vi "Read channels.vi"(8 "error in":errorcluster, 11 "Tag Bus Web Interface configuration in":refnum<class "Tag Bus Web Interface configuration.lvclass">) -> (0 "error out":errorcluster, 2 "channels":refnum<class "TBM channel.lvclass">[](array[class]), 3 "Tag Bus Web Interface configuration out":refnum<class "Tag Bus Web Interface configuration.lvclass">)   [LabVIEW 2013, in "Tag Bus Web Interface configuration.lvclass"]
uses:
  Tag Bus Web Interface configuration.lvclass
  <vilib>/NI/Tag Bus Module Framework/channel/TBM channel.lvclass
  Tag Bus Web Interface configuration.lvclass/Tag Bus Web Interface configuration.ctl
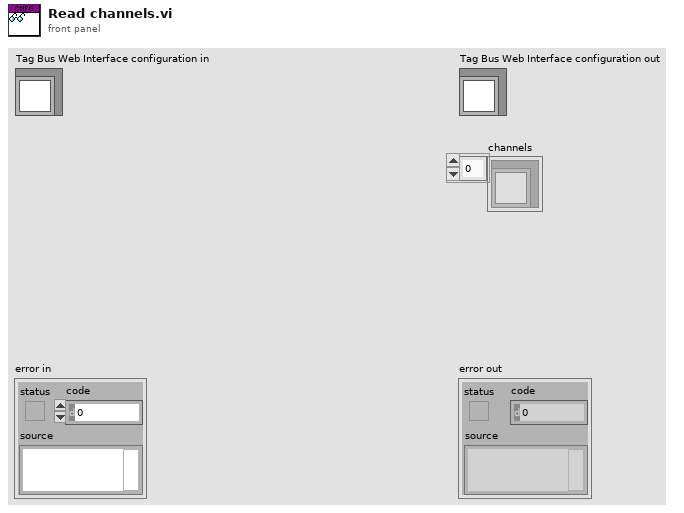
[diagram p1: front panel]
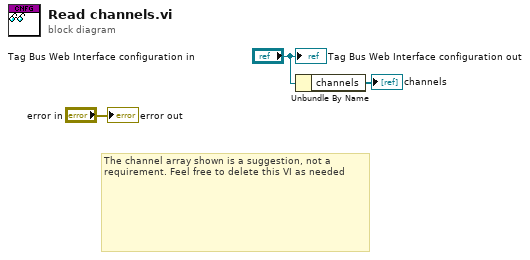
[diagram p0: block diagram]
diagram:
  # "The channel array shown is a suggestion, not a requirement. Feel free to delete this VI as needed"
  n1 = Unbundle By Name("Tag Bus Web Interface configuration in") -> ("channels"=→"channels":refnum<class "TBM channel.lvclass">[])
  "error out" <- "error in"
  "Tag Bus Web Interface configuration out" <- "Tag Bus Web Interface configuration in"
